vi "TimerReferences.vi"() -> ()   [LabVIEW 2018]
panel:
  out "timref_alarma_hmi_G6":refnum<data-value>
  out "timref_alarma_hmi_G5":refnum<data-value>
  out "timref_alarma_hmi_G4":refnum<data-value>
  out "timref_alarma_hmi_G3":refnum<data-value>
  out "timref_alarma_hmi_G2":refnum<data-value>
  out "timref_alarma_hmi_G1":refnum<data-value>
  out "timref_tol_AVG_VL_G6":refnum<data-value>
  out "timref_tol_AVG_VL_G5":refnum<data-value>
  out "timref_tol_AVG_VL_G4":refnum<data-value>
  out "timref_tol_AVG_VL_G3":refnum<data-value>
  out "timref_tol_AVG_VL_G2":refnum<data-value>
  out "timref_tol_AVG_VL_G1":refnum<data-value>
  out "timref_tol_V3_V1_G6":refnum<data-value>
  out "timref_tol_V3_V1_G5":refnum<data-value>
  out "timref_tol_V3_V1_G4":refnum<data-value>
  out "timref_tol_V3_V1_G3":refnum<data-value>
  out "timref_tol_V3_V1_G2":refnum<data-value>
  out "timref_tol_V3_V1_G1":refnum<data-value>
  out "timref_tol_V2_V3_G6":refnum<data-value>
  out "timref_tol_V2_V3_G5":refnum<data-value>
  out "timref_tol_V2_V3_G4":refnum<data-value>
  out "timref_tol_V2_V3_G3":refnum<data-value>
  out "timref_tol_V2_V3_G2":refnum<data-value>
  out "timref_tol_V2_V3_G1":refnum<data-value>
  out "timref_tol_V1_V2_G6":refnum<data-value>
  out "timref_tol_V1_V2_G5":refnum<data-value>
  out "timref_tol_V1_V2_G4":refnum<data-value>
  out "timref_tol_V1_V2_G3":refnum<data-value>
  out "timref_tol_V1_V2_G2":refnum<data-value>
  out "timref_tol_V1_V2_G1":refnum<data-value>
  out "timref_tol_frec_G6":refnum<data-value>
  out "timref_tol_frec_G5":refnum<data-value>
  out "timref_tol_frec_G4":refnum<data-value>
  out "timref_tol_frec_G3":refnum<data-value>
  out "timref_tol_frec_G2":refnum<data-value>
  out "timref_tol_frec_G1":refnum<data-value>
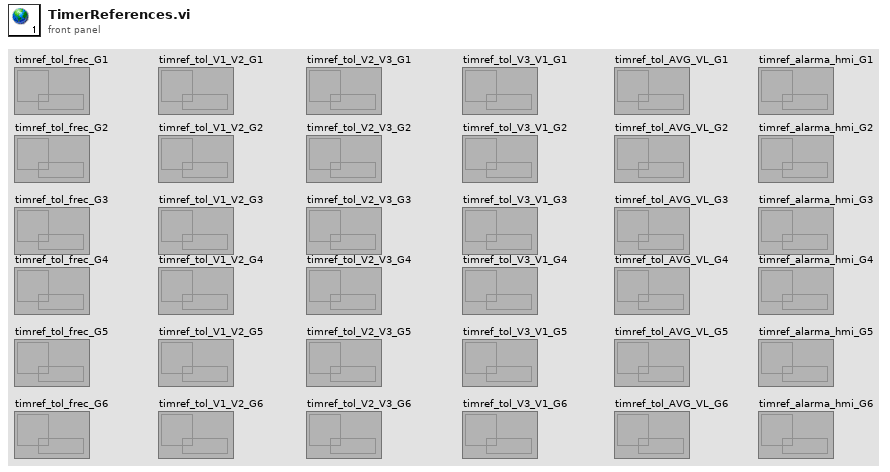
[diagram p1: front panel]
diagram:
